vi "Test_PowerRequest_Exit.vi"(8 "error in (no error)":errorcluster) -> (0 "error out":errorcluster)   [LabVIEW 2020]
doc: "Windows service power request to prevent the computer to go into hybernate if data is logged for a long time.\n\nThis routine will exit this service"
uses:
  Power Availabilty Requests/Type Defs/Power Request Type.ctl
  Power Availabilty Requests/Type Defs/Test_PR_typedef.ctl
  Power Requests.lvlib
  Builds/Sgraph_lib_V1.lvlib
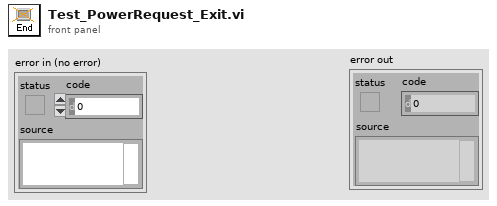
[diagram p1: front panel]
types:
  T1 = typedef "Sgraph_lib_V1.lvlib/Test_PR_typedef.ctl" = enum16{"Start-Allways-ON", "Read-handle"}
  T2 = typedef "Power Requests.lvlib/Power Request Type.ctl" = enum32{"Power Request Display Required", "Power Request System Required", "Power Request Away Mode Required", "Power Request Execution Required"}
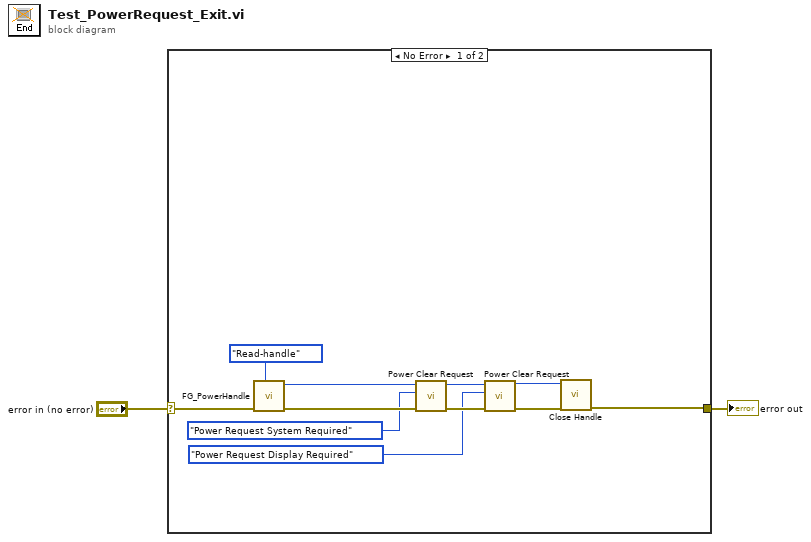
[diagram p0: block diagram]
diagram:
  n1 = case shown="No Error" "error in (no error)" {
    selector: "error in (no error)" -> [w12 w14]
    tunnel: [w3 w14] -> w1
    frame No Error {
      n2 = call "FG_PowerHandle.vi"("Enum"=Test_PR_typedef."Read-handle", "error in (no error)"=w12) -> ("error out"=w10:errorcluster, "Handle out"=w11:u32)  [unwired: 8 in]
      n3 = call "Power Clear Request.vi"("error in (no error)"=w10, "Power Request Type"=Power_Request_Type."Power Request System Required", "Handle in"=w11) -> ("error out"=w7:errorcluster, "Handle out"=w8:u32)  [unwired: 6 in, 1 out]
      n4 = call "Power Clear Request.vi"("error in (no error)"=w7, "Power Request Type"=Power_Request_Type."Power Request Display Required", "Handle in"=w8) -> ("error out"=w4:errorcluster, "Handle out"=w5:u32)  [unwired: 6 in, 1 out]
      n5 = call "Close Handle.vi"("error in (no error)"=w4, "Handle"=w5) -> ("error out"=w3:errorcluster)  [unwired: 8 in, 1 out]
    }
    frame Error {
    }
  }
  "error out" <- w1
